vi "Debug_SetMillis.vi"(8 "error in (no error)":errorcluster, 10 "Milliseconds":u32, 11 "SpinCoater in":refnum<class "SpinCoater.lvclass">) -> (0 "error out":errorcluster, 3 "SpinCoater out":refnum<class "SpinCoater.lvclass">)   [LabVIEW 2020, in "SpinCoater.lvclass"]
uses:
  <instrlib>/Classes/SpinCoater/SpinCoater.lvclass
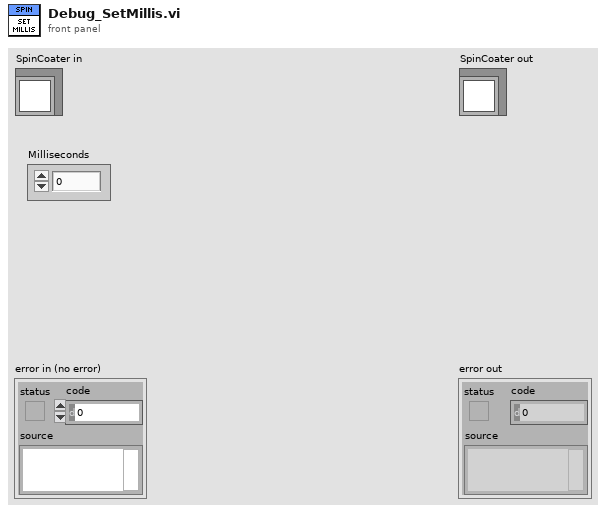
[diagram p1: front panel]
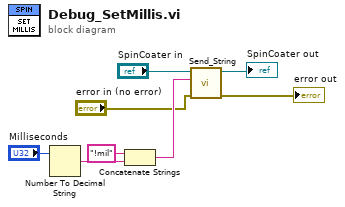
[diagram p0: block diagram]
diagram:
  n1 = Number To Decimal String(number="Milliseconds") -> (decimal integer string=w8:string)  [unwired: 1 in]
  n2 = Concatenate Strings("!mil" ("string"), w8) -> (w5:string)
  n3 = call-dynamic "Send_String.vi"("error in (no error)"="error in (no error)", "String"=w5, "SpinCoater in"="SpinCoater in") -> ("error out"=→"error out":errorcluster, "SpinCoater out"=→"SpinCoater out":refnum<class "SpinCoater.lvclass">)  [unwired: 6 in, 1 out]
